vi "User access manager GUI.vi"(8 "error in (no error)":errorcluster, 9 "Part 11?":bool, 10 "Security level":T1=10, 11 "Password Filepath":path=path "C:/Documents and Settings/default/Desktop/New Folder/passwords.log") -> (0 "error out":errorcluster)   [LabVIEW 2013]
doc: "This is a pop-up panel which lets a system supervisor (security level of 10 required to use this utility) setup up, edit and monitor user access to a system. From a custom run-time menu the supervisor can choose to:\n-Create new user\n-Activate or de-activate a user\n-Re-new privledges of a locked out or expired user\n-Delete an account\n-Configure User Access Manager properties (which are stored in the password file).\n\nIt uses a filepath to an encrypted password file. If there is a file read error a custom error code is returned (error not announced here). \n\nAll operatins performed with the User Access Manager are returned in the activity log, which can be written to an activity log file by other VIs."
uses:
  User Access Type defs/Security level U8.ctl
  GUI/GUI.lvlib
panel:
  out "activity string":string
  in  "All Users":i32(listbox)
  out "State case":string
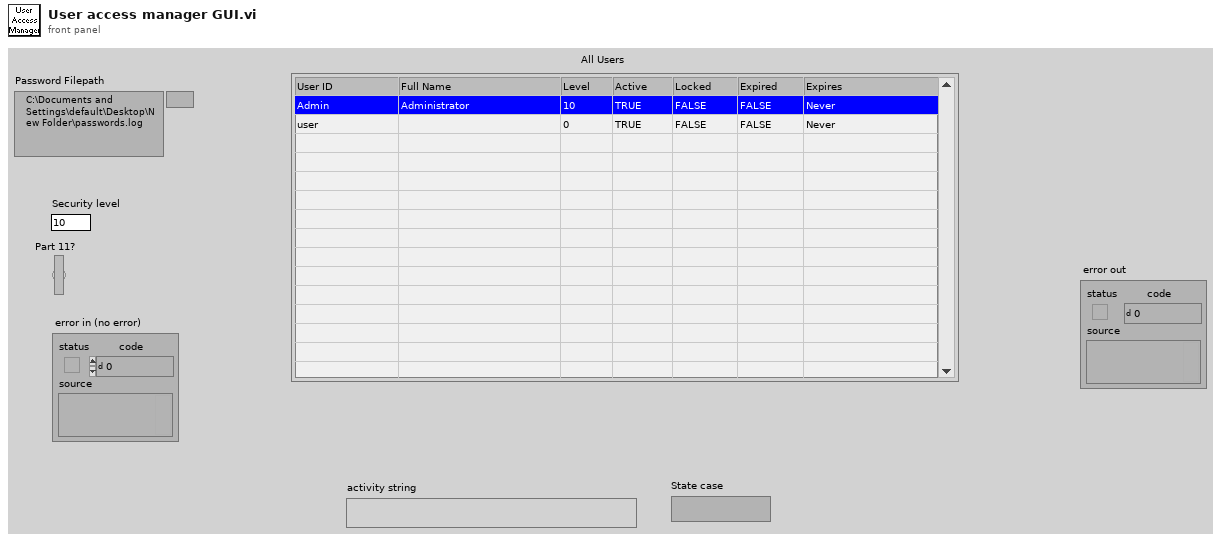
[diagram p1: front panel]
types:
  T1 = typedef "Security level U8.ctl" = u8
  T2 = enum16{"Initialize", "Write activities to file", "Write DIT", "Time to add DIT?"}
  T3 = typedef "All users access configuration cluster.ctl" = cluster{"Max ID attempts":i32, "Max password attempts":i32, "Expiration enabled":bool, "Expire days":i32, "User array":T4, "Min password char":i32}
  T4 = typedef "User access cluster array.ctl" = T5[]
  T5 = typedef "User access cluster.ctl" = cluster{"Active?":bool, "User ID":string, "Password":string, "Name":string, "Security level":T1, "Expired?":bool, "Expire sec":dbl, "Locked?":bool, "New?":bool}
  T6 = typedef "Acitivity cluster array.ctl" = T7[]
  T7 = typedef "Acitivity cluster.ctl" = cluster{"Epoch sec":dbl, "Activity":string}
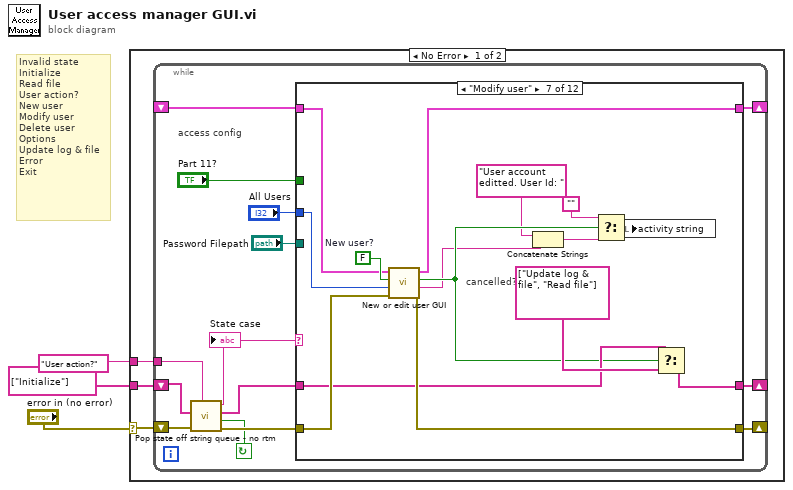
[diagram p0: block diagram]
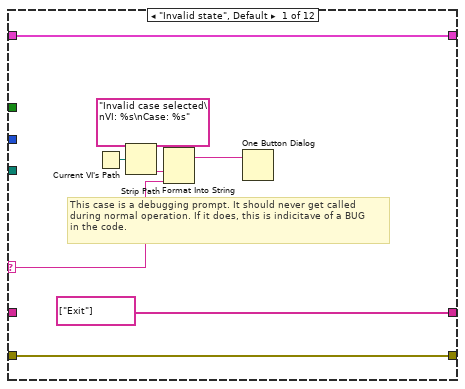
[diagram p2: hidden frame]
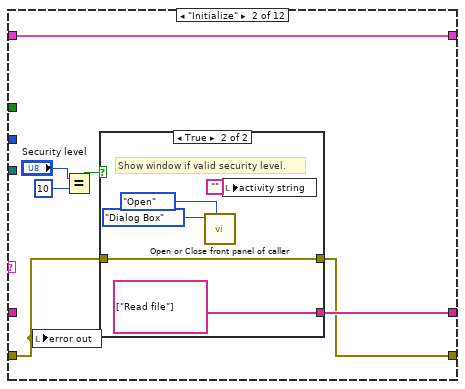
[diagram p3: hidden frame]
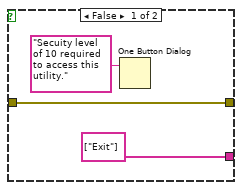
[diagram p4: hidden frame]
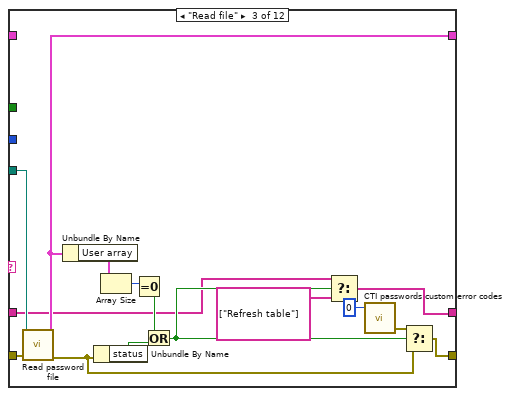
[diagram p5: hidden frame]
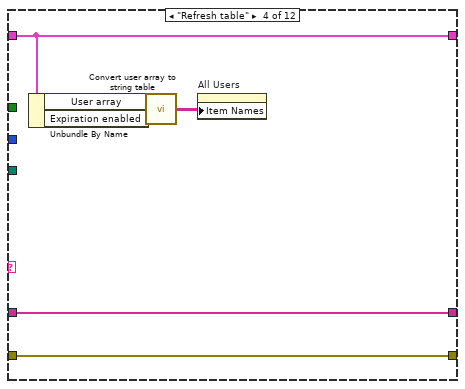
[diagram p6: hidden frame]
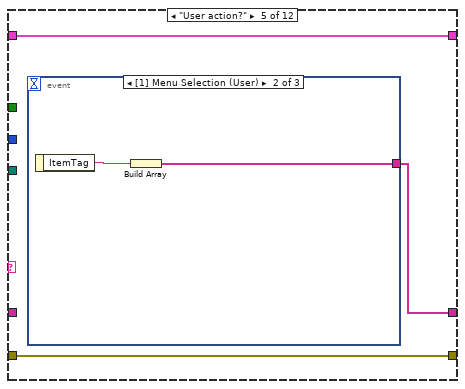
[diagram p7: hidden frame]
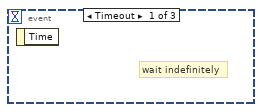
[diagram p8: hidden frame]
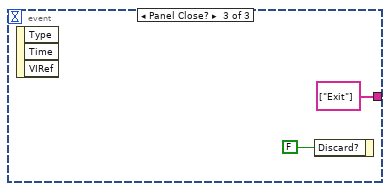
[diagram p9: hidden frame]
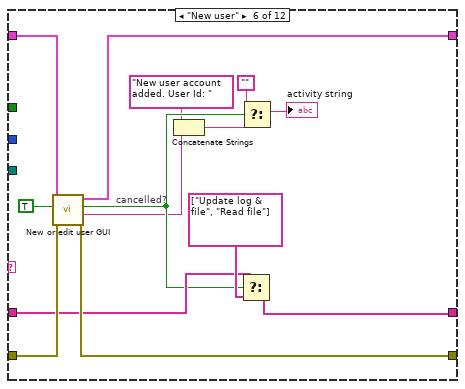
[diagram p10: hidden frame]
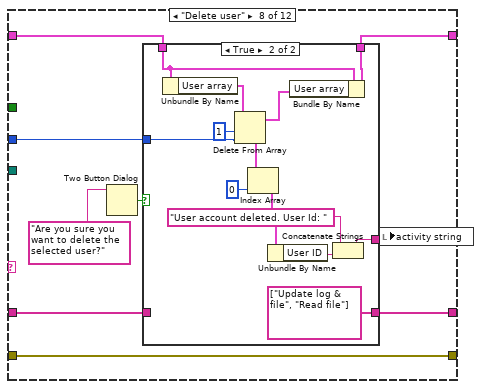
[diagram p11: hidden frame]
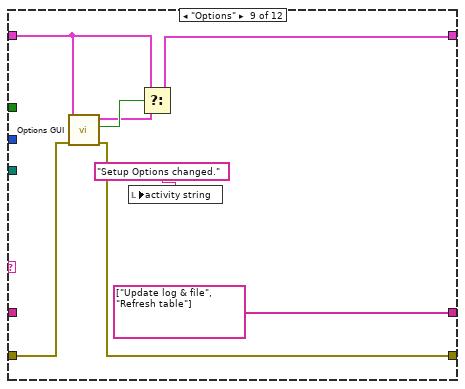
[diagram p13: hidden frame]
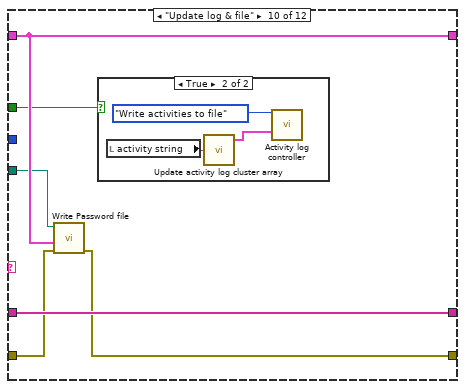
[diagram p14: hidden frame]
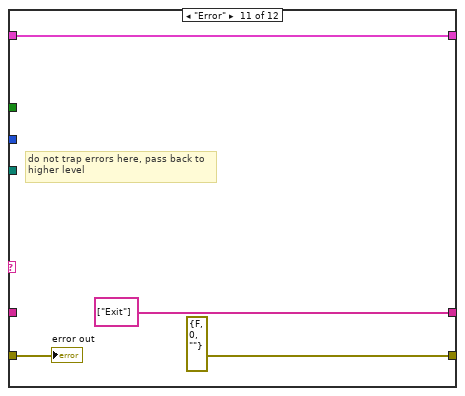
[diagram p16: hidden frame]
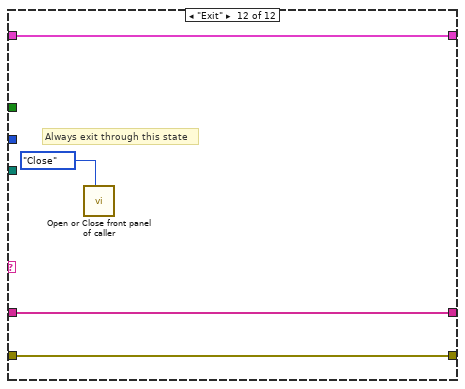
[diagram p17: hidden frame]
diagram:
  # "Invalid state\nInitialize\nRead file\nUser action?\nNew user\nModify user\nDelete user\nOptions\nUpdate log & file\nError\nExit"
  n1 = case shown="No Error" "error in (no error)" {
    selector: "error in (no error)" -> [w6 _]
    tunnel: string[] ["Initialize"] ("State que out") -> [w5 _]
    tunnel: "User action?" ("Default state") -> [w4 _]
    frame No Error {
      n2 = while {
        tunnel: w4 -> [w12]
        shift-left: w5 -> [w16]
        shift-right: [w14] -> _
        shift-left: w6 -> [w20]
        shift-right: [w18] -> _
        shift-right: [w10] -> _
        shift-left: _ -> [w11]
        stop <- w13 continue-if-true
        # "access config"
        n3 = call "Pop state off string queue - no rtm.vi"("Default state"=w12, "error in (no error)"=w20, "State que in"=w16) -> ("error out"=w19:errorcluster, "Not Exit?"=w13:bool, "State que out"=w15:string[], "State case"=w17:string)  [unwired: 5 out]
        "State case" <- w17
        n4 = case shown="\"Modify user\"" w17 {
          selector: w17 -> [w23 _ _ _ _ _ _ _ _ _ _ _]
          tunnel: [w28 w29 w52 w62 w67 w84 w99 w109 w132 w135 errorcluster {"status"=FALSE, "code"=0, "source"=""} ("error out") w149] -> w18
          tunnel: w19 -> [w28 w30 w58 w62 w67 w85 w100 w109 w133 w136 w144 w149]
          tunnel: [string[] ["Exit"] ("State que out") w35 w44 w60 w65 w80 w95 w108 string[] ["Update log & file", "Refresh table"] ("State que out") w139 string[] ["Exit"] ("State que out") w150] -> w14
          tunnel: w15 -> [_ _ w45 w60 _ w81 w96 w102 _ w139 _ w150]
          tunnel: [w21 w34 w56 w61 w66 w78 w93 w104 w128 w138 w143 w148] -> w10
          tunnel: w11 -> [w21 w34 _ w61 w66 w79 w94 w105 w129 w138 w143 w148]
          tunnel: "Password Filepath" -> [_ _ w57 _ _ _ _ _ _ w137 _ _]
          tunnel: "All Users" -> [_ _ _ _ _ _ w86 w101 _ _ _ _]
          tunnel: "Part 11?" -> [_ _ _ _ _ _ _ _ _ w134 _ _]
          frame "Invalid state", Default {
            # "This case is a debugging prompt. It should never get called\nduring normal operation. If it does, this is indicitave of a BUG\nin the code."
            n5 = Current VI's Path() -> (path=w25:path)
            n6 = Strip Path(path=w25) -> (name=w24:string)  [unwired: 1 out]
            n7 = Format Into String(format string="Invalid case selected\nVI: %s\nCase: %s" ("message"), w24, w23) -> (resulting string=w26:string)  [unwired: 2 in, 1 out]
            n8 = One Button Dialog(message=w26) -> ()  [unwired: 2 out]
          }
          frame "Initialize" {
            n9 = local write "error out"(w30) -> ()
            n10 = Equal?(x="Security level", y=T1 10) -> (x = y?=w31:bool)
            n11 = case shown="True" w31 {
              tunnel: [string[] ["Exit"] ("State que out") string[] ["Read file"] ("State que out")] -> w35
              tunnel: w30 -> [w36 w41]
              tunnel: [w36 w41] -> w29
              frame False {
                n12 = One Button Dialog(message="Secuity level of 10 required to access this utility.") -> ()  [unwired: 2 out]
              }
              frame True {
                # "Show window if valid security level."
                n13 = call "Open or Close front panel of caller.vi"("Control"=enum16{"Open", "Close", "Status", "No Change"}."Open", "Is Dialog?"=enum16{"Normal", "Dialog Box"}."Dialog Box") -> ()  [unwired: 2 in, 6 out]
                n14 = local write "activity string"("" ("activity string")) -> ()
              }
            }
          }
          frame "Read file" {
            n15 = call "Read password file.vi"("error in (no error)"=w58, "file path"=w57) -> ("error out"=w53:errorcluster, "Access Configuration"=w56:T3)  [unwired: 8 out]
            n16 = Unbundle By Name(w56) -> ("User array"=w55:T4)
            n17 = Unbundle By Name(w53) -> ("status"=w50:bool)
            n18 = Array Size(array=w55) -> (size(s)=w54:i32)
            n19 = Equal To 0?(x=w54) -> (x = 0?=w51:bool)
            n20 = Or(x=w51, y=w50) -> (x .or. y?=w46:bool)
            n21 = Select(t=w45, s=w46, f=string[] ["Refresh table"] ("State que out")) -> (s? t:f=w44:string[])
            n22 = call "CTI passwords custom error codes.vi"("error index"=0) -> ("error out"=w49:errorcluster)  [unwired: 1 in, 3 out]
            n23 = Select(t=w49, s=w46, f=w53) -> (s? t:f=w52:errorcluster)
          }
          frame "Refresh table" {
            n24 = Unbundle By Name(w61) -> ("User array"=w64:T4, "Expiration enabled"=w59:bool)
            n25 = call "Convert user array to string table.vi"("Expiration enabled"=w59, "User array"=w64) -> ("Table"=w63:string[][])  [unwired: 3 out]
            n26 = property on="All Users" class="MCListbox (strict)"("Item Names"=w63) -> ()  [unwired: 2 in, 2 out]
          }
          frame "User action?" {
            n27 = event shown="[1] Menu Selection (User)" {
              selector: _ -> [_ _ _]
              dyn-events: _ -> [_ _ _]
              timeout: _ -> [_ _ _]
              tunnel: [_ w68 string[] ["Exit"] ("State que out")] -> w65
              event Timeout {
                # "wait indefinitely"
                n28 = event-data() -> ()  [unwired: 2 out]
              }
              event Menu Selection (User) {
                n29 = event-data() -> ("ItemTag"=w69:string)  [unwired: 1 out]
                n30 = Build Array(w69) -> (w68:string[])
              }
              event Panel Close? {
                n31 = event-data() -> ()  [unwired: 4 out]
                n32 = event-data("Discard?"=FALSE) -> ()  [unwired: 1 in, 1 out]
              }
            }
          }
          frame "New user" {
            # "cancelled?"
            n33 = call "New or edit user GUI.vi"("error in (no error)"=w85, "New user?"=TRUE, "Access Configuration in"=w79) -> ("error out"=w84:errorcluster, "User ID"=w75:string, "Cancelled?"=w77:bool, "Access Configuration out"=w78:T3)  [unwired: 1 in, 4 out]
            n34 = Concatenate Strings("New user account added. User Id: ", w75) -> (w74:string)
            n35 = Select(t=w81, s=w77, f=string[] ["Update log & file", "Read file"] ("State que out")) -> (s? t:f=w80:string[])
            n36 = Select(t="", s=w77, f=w74) -> (s? t:f=→"activity string":string)
          }
          frame "Modify user" {
            w98 = FALSE  # New user?
            # "cancelled?"
            n37 = call "New or edit user GUI.vi"("error in (no error)"=w100, "Edit index"=w86, "New user?"=w98, "Access Configuration in"=w94) -> ("error out"=w99:errorcluster, "User ID"=w90:string, "Cancelled?"=w92:bool, "Access Configuration out"=w93:T3)  [unwired: 4 out]
            n38 = Concatenate Strings("User account editted. User Id: ", w90) -> (w89:string)
            n39 = Select(t="", s=w92, f=w89) -> (s? t:f=w87:string)
            n40 = local write "activity string"(w87) -> ()
            n41 = Select(t=w96, s=w92, f=string[] ["Update log & file", "Read file"] ("State que out")) -> (s? t:f=w95:string[])
          }
          frame "Delete user" {
            n42 = Two Button Dialog(message="Are you sure you want to delete the selected user?") -> (T button?=w107:bool)  [unwired: 2 out]
            n43 = case shown="True" w107 {
              tunnel: [w110 string[] ["Update log & file", "Read file"] ("State que out")] -> w108
              tunnel: w105 -> [w112 w120]
              tunnel: [w112 w119] -> w104
              tunnel: ["" w123] -> w103
              tunnel: w102 -> [w110 _]
              tunnel: w101 -> [_ w117]
              frame False {
              }
              frame True {
                n44 = Unbundle By Name(w120) -> ("User array"=w122:T4)
                n45 = Delete From Array(array=w122, length=1, index=w117) -> (deleted portion=w115:T4, array with subset deleted=w121:T4)
                n46 = Index Array(array=w115, index=0) -> (element=w113:T5)
                n47 = Unbundle By Name(w113) -> ("User ID"=w116:string)
                n48 = Bundle By Name(cluster=w120, "User array"=w121) -> (w119:T3)
                n49 = Concatenate Strings("User account deleted. User Id: ", w116) -> (w123:string)
              }
            }
            n50 = local write "activity string"(w103) -> ()
          }
          frame "Options" {
            n51 = call "Options GUI.vi"("error in (no error)"=w133, "Access Configuration in"=w129) -> ("error out"=w132:errorcluster, "Cancelled?"=w131:bool, "Access Configuration out"=w130:T3)  [unwired: 7 out]
            n52 = local write "activity string"("Setup Options changed." ("activity string")) -> ()
            n53 = Select(t=w129, s=w131, f=w130) -> (s? t:f=w128:T3)
          }
          frame "Update log & file" {
            n54 = call "Write Password file.vi"("error in (no error)"=w136, "Access Configuration"=w138, "Path"=w137) -> ("error out"=w135:errorcluster)  [unwired: 8 out]
            n55 = case shown="True" w134 {
              frame False {
              }
              frame True {
                n56 = local read "activity string"() -> (w142:string)
                n57 = call "Update activity log cluster array.vi"("Activity description"=w142) -> ("Activity log out"=w141:T6)  [unwired: 1 in, 3 out]
                n58 = call "Activity log controller.vi"("Mode"=T2."Write activities to file", "New activities"=w141) -> ()  [unwired: 4 in, 10 out]
              }
            }
          }
          frame "Error" {
            # "do not trap errors here, pass back to\nhigher level"
            "error out" <- w144
          }
          frame "Exit" {
            # "Always exit through this state"
            n59 = call "Open or Close front panel of caller.vi"("Control"=enum16{"Open", "Close", "Status", "No Change"}."Close") -> ()  [unwired: 3 in, 6 out]
          }
        }
      }
    }
    frame Error {
    }
  }
